vi "Serial.vi"() -> ()   [LabVIEW 2013]
uses:
  Serial - Settings.ctl
  <vilib>/Instr/_visa.llb/VISA Configure Serial Port (Instr).vi
panel:
  in  "串口端口选择":refnum<visa-resource-name>="COM3"
  in  "串口设置":T1={"波特率"=9600, "数据比特"=8, "奇偶"=enum."None", "停止位"=10, "流控制"=0} {"流控制" items=["无"=0, "XON/XOFF"=1, "RTS/CTS"=2, "DTR/DSR"=4]; "停止位" items=["1.0"=10, "1.5"=15, "2.0"=20]; "数据比特" min=5 max=8 step=1; "波特率" items=["75"=75, "110"=110, "134"=134, "150"=150, "300"=300, "600"=600, "1200"=1200, "1800"=1800, "2400"=2400, "4800"=4800, "7200"=7200, "9600"=9600, "14400"=14400, "19200"=19200, "28800"=28800, "38400"=38400, "56000"=56000, "57600"=57600, "115200"=115200, "128000"=128000, "230400"=230400]}
  in  "?":bool
  in  "?":bool
  in  "发送区":string
  out "接受区":string
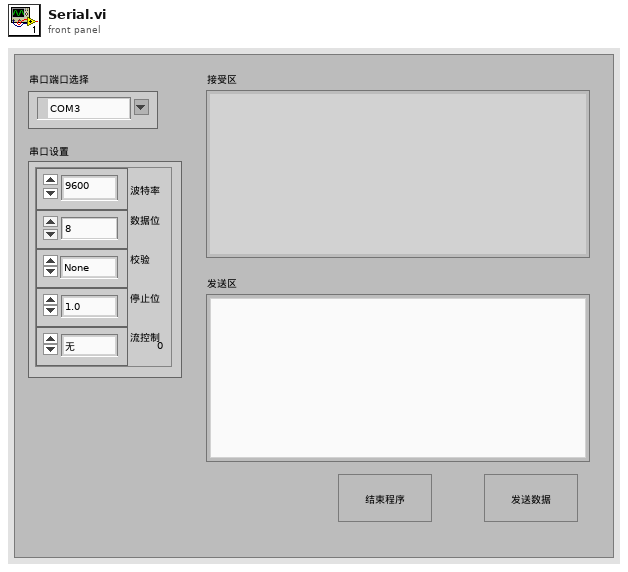
[diagram p1: front panel]
types:
  T1 = typedef "Serial - Settings.ctl" = cluster{"波特率":u32, "数据比特":u16, "奇偶":enum16{"None", "Odd", "Even", "Mark", "Space"}, "停止位":u16, "流控制":u16}
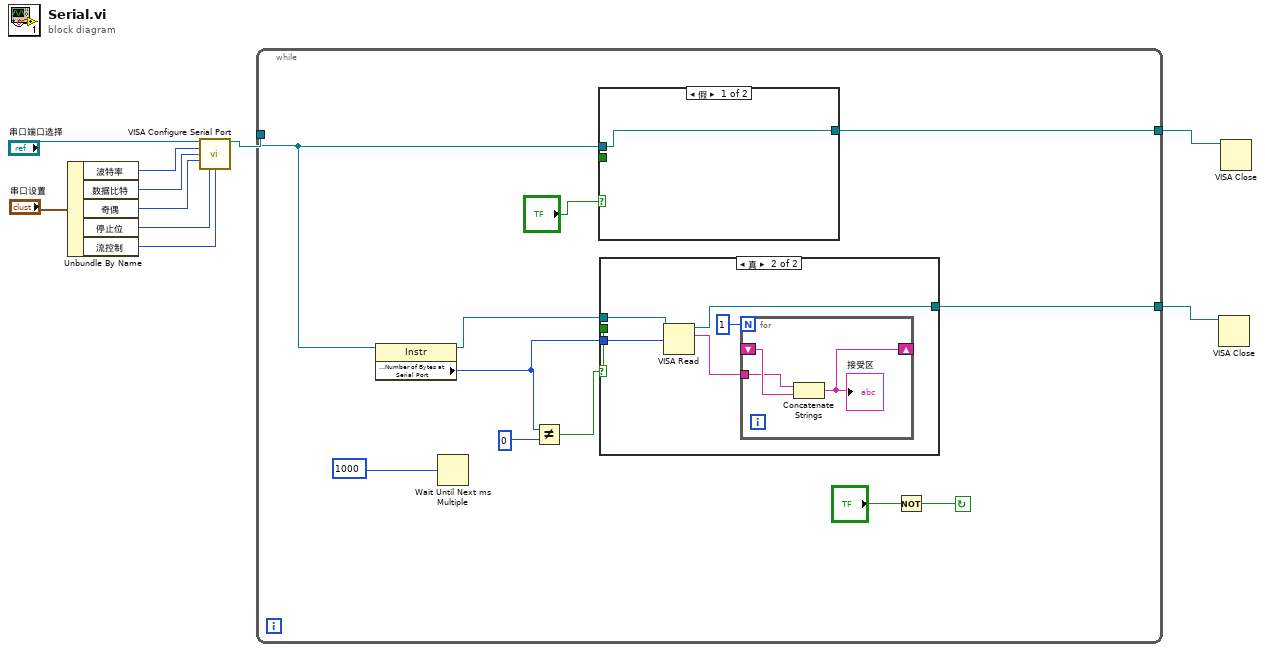
[diagram p0: block diagram]
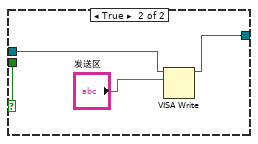
[diagram p3: hidden frame]
diagram:
  n1 = Unbundle By Name("串口设置") -> ("波特率"=w4:u32, "数据比特"=w5:u16, "奇偶"=w6:enum16{"None", "Odd", "Even", "Mark", "Space"}, "停止位"=w7:u16, "流控制"=w8:u16)
  n2 = call-poly "VISA Configure Serial Port"("VISA resource name"="串口端口选择", "baud rate (9600)"=w4, "data bits (8)"=w5, "parity (0:none)"=w6, "stop bits (10: 1 bit)"=w7, "flow control (0:none)"=w8) -> ("VISA resource name out"=w2:refnum<visa-resource-name>)  [unwired: 3 in, 6 out]
  n3 = while {
    tunnel: [w19] -> w10
    tunnel: [w18] -> w9
    tunnel: w2 -> [w14]
    stop <- w13 continue-if-true
    n4 = property class="Instr"(reference=w14) -> (reference out=w12:refnum<visa-resource-name>, "Serial Settings:Number of Bytes at Serial Port"=w16:u32)  [unwired: 1 in, 1 out]
    n5 = Wait Until Next ms Multiple(millisecond multiple=1000) -> ()  [unwired: 1 out]
    n6 = Not Equal?(x=w16, y=0) -> (x != y?=w15:bool)
    n7 = case shown="假" "?" {
      selector: "?" -> [_ w36]
      tunnel: [_ w36] -> _
      tunnel: w14 -> [w32 w34]
      tunnel: [w32 w33] -> w19
      frame False {
      }
      frame True {
        n8 = VISA Write(VISA resource name=w34, write buffer="发送区") -> (VISA resource name out=w33:refnum<visa-resource-name>)  [unwired: 1 in, 2 out]
      }
    }
    n9 = case shown="真" w15 {
      selector: w15 -> [_ w24]
      tunnel: w12 -> [w22 w27]
      tunnel: [w22 w26] -> w18
      tunnel: w16 -> [_ w25]
      tunnel: [_ w24] -> _
      frame False {
      }
      frame True {
        n10 = VISA Read(VISA resource name=w27, byte count=w25) -> (VISA resource name out=w26:refnum<visa-resource-name>, read buffer=w28:string)  [unwired: 1 in, 2 out]
        n11 = for {
          N: 1 -> [_]
          tunnel: w28 -> [w30]
          shift-right: [w29] -> _
          shift-left: _ -> [w31]
          n12 = Concatenate Strings(w30, w31) -> (w29:string)
          "接受区" <- w29
        }
      }
    }
    n13 = Not(x="?") -> (.not. x?=w13:bool)
  }
  n14 = VISA Close(VISA resource name=w9) -> ()  [unwired: 1 in, 1 out]
  n15 = VISA Close(VISA resource name=w10) -> ()  [unwired: 1 in, 1 out]
